vi "Redo.vi"(8 "error in (no error)":errorcluster, 11 "All Queue in":T2) -> (0 "error out":errorcluster, 2 "Ctrl Val.Get All":T1[](array[typedef]), 3 "All Queue out":T2, 4 "Redo Enable":bool, 6 "Undo Enable":bool)   [LabVIEW 2015, in "UndoLibrary.lvlib"]
doc: "This VI stores the values to perform the redo action."
uses:
  UndoLibrary.lvlib
  Controls/cluster_All Queue.ctl
  Controls/cluster_Control Value.ctl
  QueueOperations/QueueOperations.lvlib
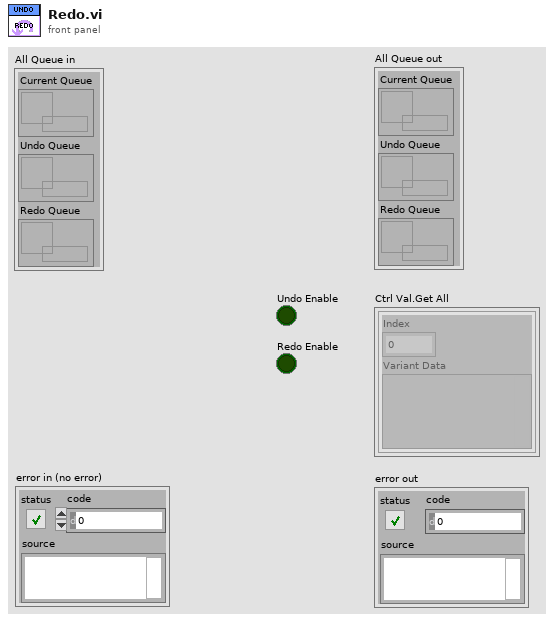
[diagram p1: front panel]
types:
  T1 = typedef "UndoLibrary.lvlib/cluster_Control Value.ctl" = cluster{"Index":i32, "Variant Data":variant}
  T2 = typedef "UndoLibrary.lvlib/cluster_All Queue.ctl" = cluster{"Current Queue":refnum<queue>, "Undo Queue":refnum<queue>, "Redo Queue":refnum<queue>}
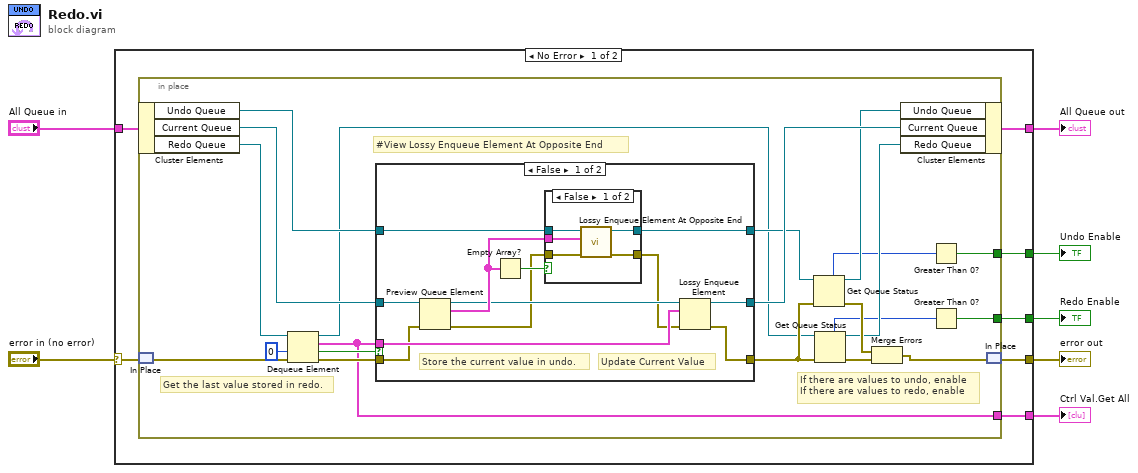
[diagram p0: block diagram]
diagram:
  n1 = case shown="No Error" "error in (no error)" {
    selector: "error in (no error)" -> [w13 w59]
    tunnel: [w12 w59] -> w7
    tunnel: "All Queue in" -> [w11 w58]
    tunnel: [w14 _] -> w4
    tunnel: [w10 w58] -> w3
    tunnel: [w9 _] -> w2
    tunnel: [w8 _] -> w1
    frame No Error {
      n2 = in-place {
        in-place-border: [w32] -> w14
        in-place-border: [w17] -> w9
        in-place-border: [w15] -> w8
        # "Get the last value stored in redo."
        # "If there are values to undo, enable\nIf there are values to redo, enable"
        # "#View Lossy Enqueue Element At Opposite End"
        n3 = in-place-cluster #1(w11) -> ("Undo Queue"=w30:refnum<queue>, "Current Queue"=w29:refnum<queue>, "Redo Queue"=w28:refnum<queue>)
        n4 = in-place-match #2(w13) -> (w31:errorcluster)
        n5 = Dequeue Element(queue=w28, timeout in ms (-1)=0, error in (no error)=w31) -> (queue out=w20:refnum<queue>, element=w32:T1[], timed out?=w34:bool, error out=w35:errorcluster)
        n6 = case shown="False" w34 {
          tunnel: w30 -> [w47 w57]
          tunnel: [w46 w57] -> w24
          tunnel: w35 -> [w38 w55]
          tunnel: w32 -> [w41 _]
          tunnel: w29 -> [w44 w56]
          tunnel: [w40 w56] -> w27
          tunnel: [w39 w55] -> w22
          frame False {
            # "Store the current value in undo."
            # "Update Current Value"
            n7 = Preview Queue Element(queue=w44, error in (no error)=w38) -> (queue out=w42:refnum<queue>, element=w43:T1[], error out=w37:errorcluster)  [unwired: 1 in, 1 out]
            n8 = Empty Array?(array=w43) -> (empty?=w45:bool)
            n9 = case shown="False" w45 {
              tunnel: w47 -> [w52 w53]
              tunnel: [w48 w53] -> w46
              tunnel: [w49 w54] -> w36
              tunnel: w37 -> [w50 w54]
              tunnel: w43 -> [w51 _]
              frame False {
                n10 = call "Lossy Enqueue Element At Opposite End.vi"("error in (no error)"=w50, "element"=w51, "queue in"=w52) -> ("error out"=w49:errorcluster, "queue out"=w48:refnum<queue>)  [unwired: 5 in, 2 out]
              }
              frame True {
              }
            }
            n11 = Lossy Enqueue Element(queue=w42, element=w41, error in (no error)=w36) -> (queue out=w40:refnum<queue>, error out=w39:errorcluster)  [unwired: 2 out]
          }
          frame True {
          }
        }
        n12 = Get Queue Status(queue=w24, error in (no error)=w22) -> (queue out=w23:refnum<queue>, error out=w25:errorcluster, # elements in queue=w18:i32)  [unwired: 1 in, 5 out]
        n13 = Get Queue Status(queue=w20, error in (no error)=w22) -> (queue out=w19:refnum<queue>, error out=w26:errorcluster, # elements in queue=w16:i32)  [unwired: 1 in, 5 out]
        n14 = Merge Errors(w25, w26) -> (w21:errorcluster)
        n15 = in-place-cluster #1("Undo Queue"=w23, "Current Queue"=w27, "Redo Queue"=w19) -> (w10:T2)
        n16 = Greater Than 0?(x=w18) -> (x > 0?=w17:bool)
        n17 = Greater Than 0?(x=w16) -> (x > 0?=w15:bool)
        n18 = in-place-match #2(w21) -> (w12:errorcluster)
      }
    }
    frame Error {
    }
  }
  "error out" <- w7
  "Ctrl Val.Get All" <- w4
  "All Queue out" <- w3
  "Undo Enable" <- w2
  "Redo Enable" <- w1
